vi "Rectangel GetRectCornerPoints.vi"(0 "bounds":T2 {"height" format="%.2f"; "width" format="%.2f"; "y" format="%.2f"; "x" format="%.2f"}, 5 "error in (no error)":errorcluster) -> (15 "X,Y":T1 {"y" format="%.2f"; "x" format="%.2f"}, 16 "X+W,Y":T1 {"y" format="%.2f"; "x" format="%.2f"}, 17 "X,Y+H":T1 {"y" format="%.2f"; "x" format="%.2f"}, 18 "X+W,Y+H":T1 {"y" format="%.2f"; "x" format="%.2f"}, 19 "error out":errorcluster)   [LabVIEW 2020]
doc: "contains"
uses:
  <resource>/Framework/Providers/Open_GDS/UML/General/Point/Point Point2D.ctl
  <resource>/Framework/Providers/Open_GDS/UML/General/Rectangle/Rectangle Rectangle2D.ctl
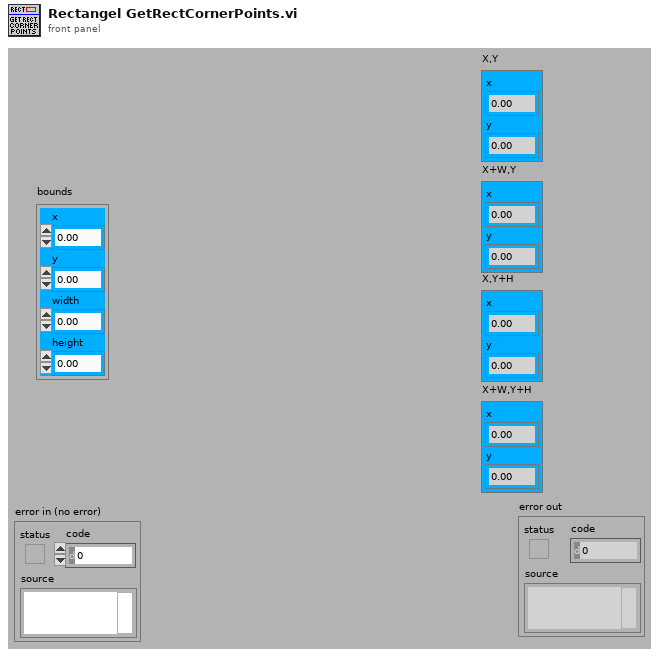
[diagram p1: front panel]
types:
  T1 = typedef "Point Point2D.ctl" = cluster{"x":dbl, "y":dbl}
  T2 = typedef "Rectangle Rectangle2D.ctl" = cluster{"x":dbl, "y":dbl, "width":dbl, "height":dbl}
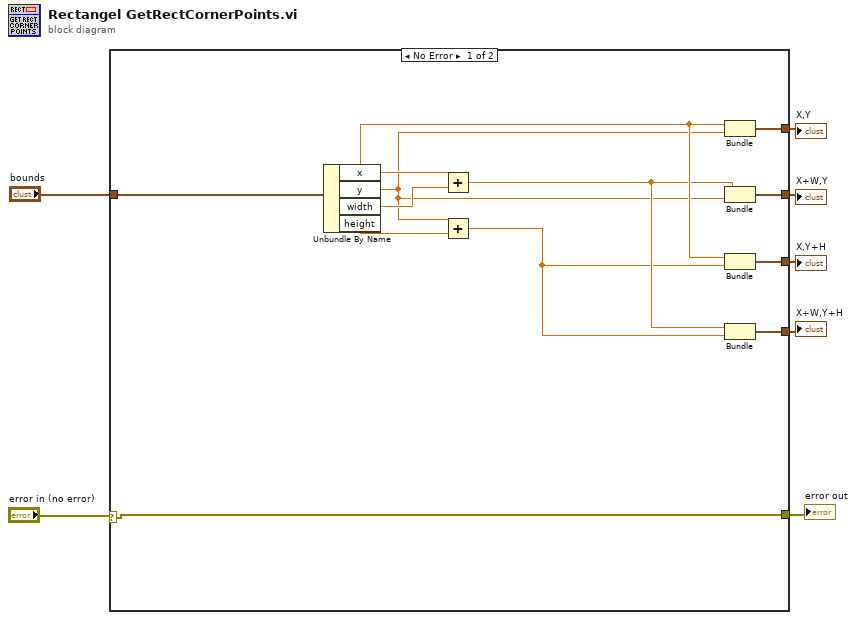
[diagram p0: block diagram]
diagram:
  n1 = case shown="No Error" "error in (no error)" {
    selector: "error in (no error)" -> [w16 w20]
    tunnel: [w16 w20] -> w7
    tunnel: "bounds" -> [w19 _]
    tunnel: [w15 _] -> w4
    tunnel: [w14 _] -> w3
    tunnel: [w13 _] -> w2
    tunnel: [w12 _] -> w1
    frame No Error {
      n2 = Unbundle By Name(w19) -> ("x"=w11:dbl, "y"=w9:dbl, "width"=w18:dbl, "height"=w17:dbl)
      n3 = Add(x=w11, y=w18) -> (x+y=w10:dbl)
      n4 = Add(x=w9, y=w17) -> (x+y=w8:dbl)
      n5 = Bundle("x"=w11, "y"=w9) -> (w15:cluster{"x":dbl, "y":dbl})  [unwired: 1 out]
      n6 = Bundle(w10, "y"=w9) -> (w12:cluster{dbl, "y":dbl})  [unwired: 1 out]
      n7 = Bundle("x"=w11, w8) -> (w14:cluster{"x":dbl, dbl})  [unwired: 1 out]
      n8 = Bundle(w10, w8) -> (w13:cluster{dbl, dbl})  [unwired: 1 out]
    }
    frame Error {
    }
  }
  "error out" <- w7
  "X+W,Y" <- w1
  "X,Y+H" <- w3
  "X+W,Y+H" <- w2
  "X,Y" <- w4
